vi "RTTERMINAL Start.vi"(11 "Control block address [hex]":u32 format="%08x") -> (3 "function return":i32)   [LabVIEW 2011, in "JLinkARM.lvlib"]
uses:
  Lib/JLinkARM.lvlib
  JLinkARM.dll
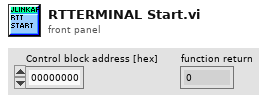
[diagram p1: front panel]
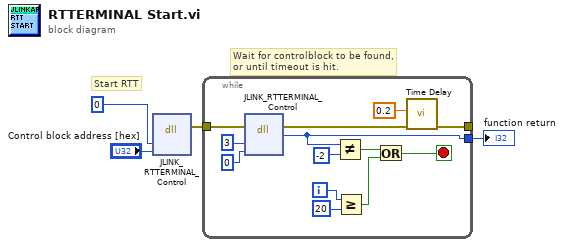
[diagram p0: block diagram]
diagram:
  # "Wait for controlblock to be found,\nor until timeout is hit."
  # "Start RTT"
  n1 = dll-call lib="C:/Documents and Settings/Anybody/Desktop/JLink_SDK_V684a/JLinkARM.*" fn="JLINK_RTTERMINAL_Control"("Cmd"=u32 0, "pRTT"="Control block address [hex]") -> (error out=w3:errorcluster)  [unwired: 6 in, 1 out]
  n2 = while {
    tunnel: w3 -> [w15]
    tunnel: [w6] -> w2
    tunnel: [w5] -> _
    i -> [w13]
    stop <- w12 stop-if-true
    n3 = dll-call lib="C:/Documents and Settings/Anybody/Desktop/JLink_SDK_V684a/JLinkARM.*" fn="JLINK_RTTERMINAL_Control"(error in=w15, "Cmd"=u32 3, "pRTT"=u32 0) -> (error out=w7:errorcluster, "return type"=w6:i32)  [unwired: 4 in, 1 out]
    n4 = Not Equal?(x=w6, y=-2) -> (x != y?=w11:bool)
    n5 = Greater Or Equal?(x=w13, y=20) -> (x >= y?=w10:bool)
    n6 = Or(x=w11, y=w10) -> (x .or. y?=w12:bool)
    n7 = call "Time Delay"("error in (no error)"=w7, "Delay Time (s)"=0.2) -> ("error out"=w5:errorcluster)  [unwired: 9 in]
  }
  "function return" <- w2
